vi "Register MQTT Client Events.vi"(8 "error in":errorcluster, 9 "MQTT Public Events":T1, 10 "Client Public Events":T2) -> (0 "error out":errorcluster)   [LabVIEW 2024, in "MQTTClient.lvlib"]
doc: "Registers the MQTT Client Events.\n_____\nCreated using DQMH Event Scripter 7.0.1.1316."
uses:
  MQTTClient.lvlib
  <vilib>/LabVIEW Open Source Project/MQTT Client/Client class/Public Events -- cluster.ctl
  <vilib>/LabVIEW Open Source Project/MQTT Control Packets/Control Packets/CONNACK/Connect Return Code -- enum.ctl
  <vilib>/LabVIEW Open Source Project/MQTT Control Packets/Control Packets/PUBLISH/PUBLISH.lvclass
  <vilib>/LabVIEW Open Source Project/MQTT Connection/MQTT_Base/Base Class/Public Events -- cluster.ctl
  Register MQTT Client Events Argument--cluster.ctl
  <vilib>/LabVIEW Open Source Project/MQTT Connection/MQTT_Base/Base Class/MQTT_Base.lvclass
  <vilib>/LabVIEW Open Source Project/MQTT Control Packets/Control Packets/CONNACK/CONNACK.lvclass
  <vilib>/LabVIEW Open Source Project/MQTT Client/Client class/Client.lvclass
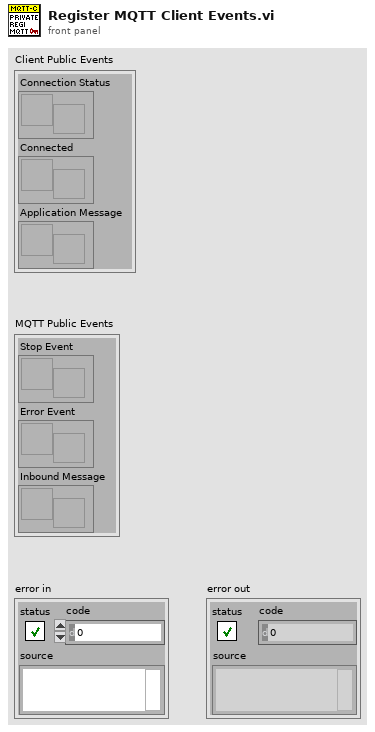
[diagram p1: front panel]
types:
  T1 = typedef "MQTT Base.lvlib/MQTT_Base.lvclass/Public Events -- cluster.ctl" = cluster{"Stop Event":refnum<user-event>, "Error Event":refnum<user-event>, "Inbound Message":refnum<user-event>}
  T2 = typedef "MQTT Client.lvlib/Client.lvclass/Public Events -- cluster.ctl" = cluster{"Connection Status":refnum<user-event>, "Connected":refnum<user-event>, "Application Message":refnum<user-event>}
  T3 = typedef "MQTTClient.lvlib/Register MQTT Client Events Argument--cluster.ctl" = cluster{"Client Public Events":T2, "MQTT Public Events":T1}
  T4 = typedef "MQTTClient.lvlib/Request Events--cluster.ctl" = cluster{"Stop Module":refnum<user-event>, "Show Panel":refnum<user-event>, "Hide Panel":refnum<user-event>, "Get Module Execution Status":refnum<user-event>, "Show Diagram":refnum<user-event>, "Change Panel":refnum<user-event>, "Initialise Connection":refnum<user-event>, "Ping Connection":refnum<user-event>, "Publish to MQTT Topic":refnum<user-event>, "Close Connection":refnum<user-event>, "Connect to MQTT Server":refnum<user-event>, "Private":cluster{"Reset Ping Helper Loop Timeout":refnum<user-event>, "Sleep Ping Helper Loop":refnum<user-event>, "Register MQTT Client Events":refnum<user-event>}, "Subscribe to MQTT Topic":refnum<user-event>, "Launch":refnum<user-event>, "Private.Wake Connection Helper Loop":refnum<user-event>}
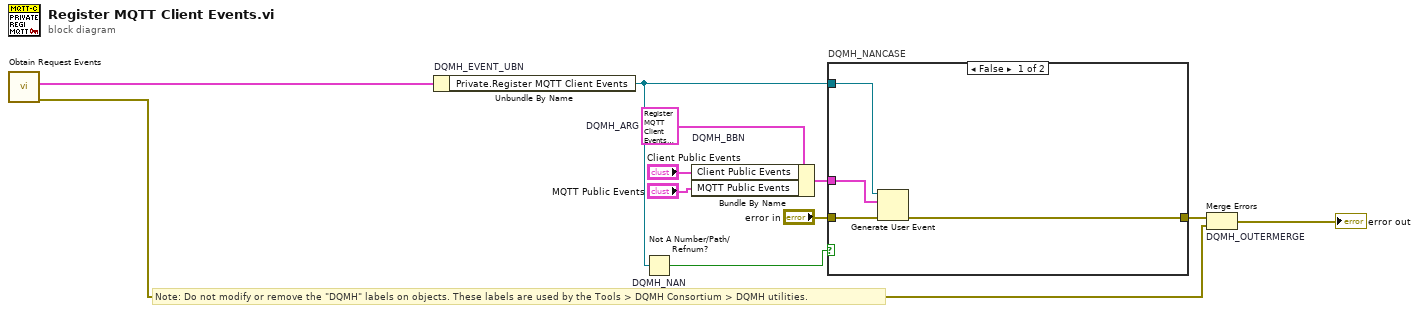
[diagram p0: block diagram]
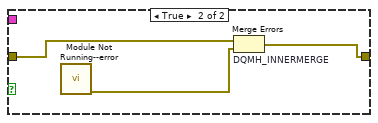
[diagram p2: hidden frame]
diagram:
  w5 = T3 {"Client Public Events"={"Connection Status"=refnum, "Connected"=refnum, "Application Message"=refnum}, "MQTT Public Events"={"Stop Event"=refnum, "Error Event"=refnum, "Inbound Message"=refnum}}  # DQMH_ARG
  # "Note: Do not modify or remove the \"DQMH\" labels on objects. These labels are used by the Tools > DQMH Consortium > DQMH utilities."
  n1 = call "Obtain Request Events.vi"() -> ("error out"=w2:errorcluster, "MQTTClient Request Events"=w1:T4)  [unwired: 10 in]
  n2 = Unbundle By Name "DQMH_EVENT_UBN"(w1) -> ("Private.Register MQTT Client Events"=w7:refnum<user-event>)
  n3 = Not A Number/Path/Refnum? "DQMH_NAN"(number/path/refnum=w7) -> (NaN/Path/Refnum?=w8:bool)
  n4 = Bundle By Name "DQMH_BBN"(cluster=w5, "Client Public Events"="Client Public Events", "MQTT Public Events"="MQTT Public Events") -> (w9:T3)
  n5 = case "DQMH_NANCASE" shown="False" w8 {
    tunnel: "error in" -> [w15 w18]
    tunnel: [w14 w17] -> w6
    tunnel: w7 -> [w13 _]
    tunnel: w9 -> [w12 _]
    frame False {
      n6 = Generate User Event(user event=w13, event data cluster=w12, error in=w15) -> (error out=w14:errorcluster)  [unwired: 1 in, 1 out]
    }
    frame True {
      n7 = call "Module Not Running--error.vi"() -> ("error out"=w16:errorcluster)  [unwired: 11 in]
      n8 = Merge Errors "DQMH_INNERMERGE"(w18, w16) -> (w17:errorcluster)
    }
  }
  n9 = Merge Errors "DQMH_OUTERMERGE"(w6, w2) -> (→"error out":errorcluster)
